vi "超标留样启动.vi"(8 "error in (no error)":errorcluster) -> (0 "error out":errorcluster)   [LabVIEW 2016, in "科盛超标留样.lvlib"]
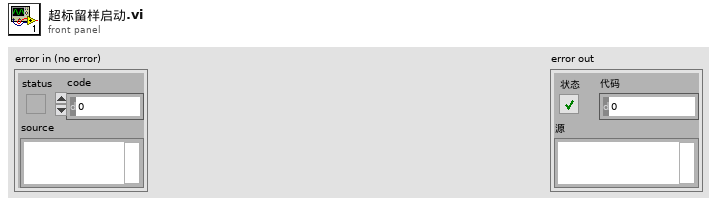
[diagram p1: front panel]
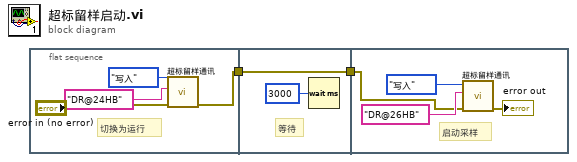
[diagram p0: block diagram]
diagram:
  n1 = flat-sequence {
    tunnel: [w3] -> w1
    tunnel: [w7] -> w2
    tunnel: w1 -> [w7]
    tunnel: w2 -> [w10]
    frame #0 {
      # "切换为运行"
      n2 = call "超标留样通讯.vi"("error in (no error)"="error in (no error)", "写入缓冲区"="DR@24HB", "功能输入"=enum16{"打开串口", "写入", "读取", "关闭串口"}."写入") -> ("error out"=w3:errorcluster)  [unwired: 6 in, 2 out]
    }
    frame #1 {
      # "等待"
      n3 = Wait (ms)(milliseconds to wait=u32 3000 ("等待时间（毫秒）")) -> ()  [unwired: 1 out]
    }
    frame #2 {
      # "启动采样"
      n4 = call "超标留样通讯.vi"("error in (no error)"=w10, "写入缓冲区"="DR@26HB", "功能输入"=enum16{"打开串口", "写入", "读取", "关闭串口"}."写入") -> ("error out"=→"error out":errorcluster)  [unwired: 6 in, 2 out]
    }
  }
